vi "多标尺的波形图表.vi"() -> ()   [LabVIEW 2010]
uses:
  <vilib>/Analysis/NI_AALBase.lvlib
panel:
  out "波形图表 2":cluster{dbl, dbl}[](graph)
  out "波形图表":cluster{dbl, dbl}[](graph)
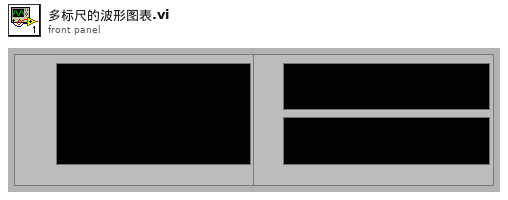
[diagram p1: front panel]
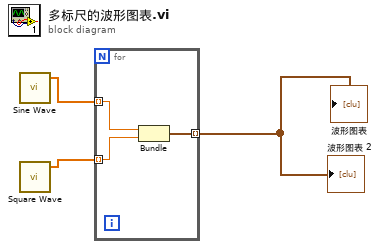
[diagram p0: block diagram]
diagram:
  n1 = call <vilib>:"Sine Wave.vi"() -> ("sine wave"=w3:dbl[])  [unwired: 5 in, 2 out]
  n2 = call <vilib>:"Square Wave.vi"() -> ("square wave"=w1:dbl[])  [unwired: 6 in, 2 out]
  n3 = for {
    tunnel: w3 -> [w6] mode=indexing
    tunnel: w1 -> [w5] mode=indexing
    tunnel: [w4] -> w2 mode=indexing
    n4 = Bundle(w6, w5) -> (w4:cluster{dbl, dbl})  [unwired: 1 in]
  }
  "波形图表" <- w2
  "波形图表 2" <- w2
